vi "get_wl.vi"() -> ()   [LabVIEW 2017, in "radiant.lvlib"]
doc: "<B>Laser Goto with FCU</B> VI tunes laser to the position <B>Wavenumber (1/cm)</B>. FCU1 is adjusted accordingly."
uses:
  <vilib>/Instr/_visa.llb/VISA Configure Serial Port (Instr).vi
  radiant.lvlib
panel:
  in  "error in (no error)":errorcluster
  out "bytes":u32
  out "fundamental (nm)":dbl format="%#_8g"
  out "VISA resource name out":refnum<visa-resource-name>
  out "error out":errorcluster
  in  "VISA resource name":refnum<visa-resource-name>="COM9"
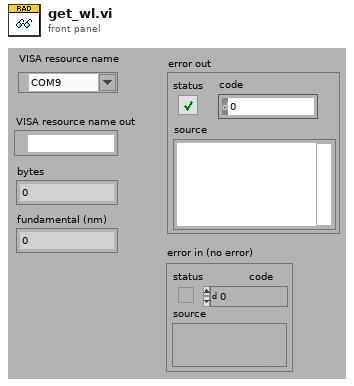
[diagram p1: front panel]
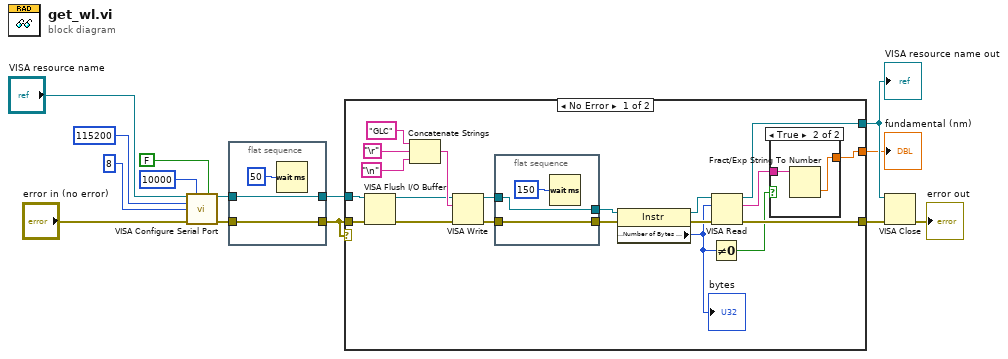
[diagram p0: block diagram]
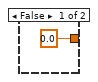
[diagram p2: hidden frame]
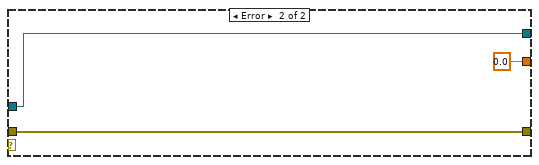
[diagram p3: hidden frame]
diagram:
  n1 = call-poly "VISA Configure Serial Port"("VISA resource name"="VISA resource name", "timeout (10sec)"=u32 10000, "Enable Termination\nChar (T)"=FALSE ("Enable Termination\nChar (T)"), "baud rate (9600)"=u32 115200, "data bits (8)"=u16 8, "error in (no error)"="error in (no error)") -> ("VISA resource name out"=w4:refnum<visa-resource-name>, "error out"=w2:errorcluster)  [unwired: 8 in]
  n2 = flat-sequence {
    tunnel: w4 -> [w17]
    tunnel: [w17] -> w3
    tunnel: w2 -> [w16]
    tunnel: [w16] -> w1
    frame #0 {
      n3 = Wait (ms)(milliseconds to wait=u32 50) -> ()  [unwired: 1 out]
    }
  }
  n4 = case shown="No Error" w1 {
    tunnel: w1 -> [w33 w46]
    tunnel: w3 -> [w32 w45]
    tunnel: [w29 w46] -> w10
    tunnel: [w28 w45] -> w9
    tunnel: [w27 0.0] -> w8
    frame No Error {
      n5 = VISA Flush I/O Buffer(VISA resource name=w32, error in (no error)=w33) -> (VISA resource name out=w31:refnum<visa-resource-name>, error out=w30:errorcluster)  [unwired: 1 in]
      n6 = Concatenate Strings("GLC" ("write"), "\r", "\n") -> (w34:string)
      n7 = VISA Write(VISA resource name=w31, write buffer=w34, error in (no error)=w30) -> (VISA resource name out=w21:refnum<visa-resource-name>, error out=w20:errorcluster)  [unwired: 1 out]
      n8 = flat-sequence {
        tunnel: w21 -> [w40]
        tunnel: [w40] -> w18
        tunnel: w20 -> [w39]
        tunnel: [w39] -> w19
        frame #0 {
          n9 = Wait (ms)(milliseconds to wait=u32 150) -> ()  [unwired: 1 out]
        }
      }
      n10 = property class="Instr"(reference=w18, error in=w19) -> (reference out=w26:refnum<visa-resource-name>, error out=w25:errorcluster, "Serial Settings:Number of Bytes at Serial Port"=w24:u32)
      "bytes" <- w24
      n11 = Not Equal To 0?(x=w24) -> (x != 0?=w23:bool)
      n12 = VISA Read(VISA resource name=w26, byte count=w24, error in (no error)=w25) -> (VISA resource name out=w28:refnum<visa-resource-name>, read buffer=w22:string, error out=w29:errorcluster)  [unwired: 1 out]
      n13 = case shown="True" w23 {
        tunnel: [0.0 w43] -> w27
        tunnel: w22 -> [_ w42]
        frame False {
        }
        frame True {
          n14 = Fract/Exp String To Number(string=w42) -> (number=w43:dbl)  [unwired: 3 in, 1 out]
        }
      }
    }
    frame Error {
    }
  }
  "VISA resource name out" <- w9
  "fundamental (nm)" <- w8
  n15 = VISA Close(VISA resource name=w9, error in (no error)=w10) -> (error out=→"error out":errorcluster)
